vi "Poly-fit-3 section.vi"(0 "2nd stage position (um)":dbl[](array[numeric]), 1 "1st stage position (um)":dbl[](array[numeric]), 2 "3rd stage position (um)":dbl[](array[numeric]), 3 "3rd QPD signal (V)":dbl[](array[numeric]), 4 "1st QPD signal (V)":dbl[](array[numeric]), 5 "2nd QPD signal (V)":dbl[](array[numeric])) -> (6 "1st Best stage position":dbl[](array[numeric]), 7 "2nd Best stage position":dbl[](array[numeric]), 8 "3rd Best stage position":dbl[](array[numeric]))   [LabVIEW 2014]
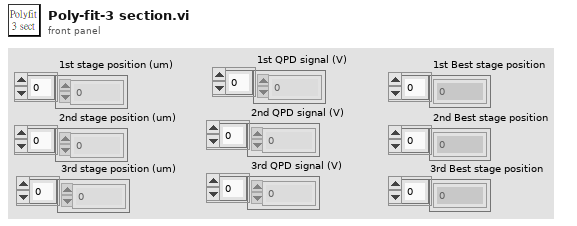
[diagram p1: front panel]
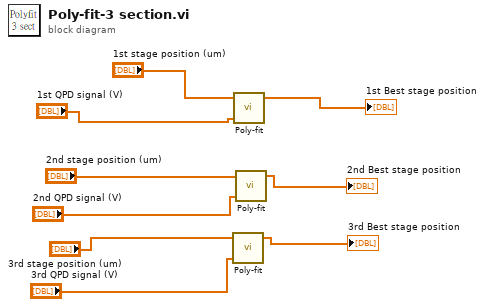
[diagram p0: block diagram]
diagram:
  n1 = call "Poly-fit.vi"("QPD signal (V)"="3rd QPD signal (V)", "stage position (um)"="3rd stage position (um)") -> ("Best stage position"=→"3rd Best stage position":dbl[])  [unwired: 2 in, 1 out]
  n2 = call "Poly-fit.vi"("QPD signal (V)"="1st QPD signal (V)", "stage position (um)"="1st stage position (um)") -> ("Best stage position"=→"1st Best stage position":dbl[])  [unwired: 2 in, 1 out]
  n3 = call "Poly-fit.vi"("QPD signal (V)"="2nd QPD signal (V)", "stage position (um)"="2nd stage position (um)") -> ("Best stage position"=→"2nd Best stage position":dbl[])  [unwired: 2 in, 1 out]
